vi "Configure Event Search.vi"   [LabVIEW 2010, in "Agilent 2000 3000 X-Series.lvlib"]
doc: "Configures the event search."
uses:
  <instrlib>/Agilent 2000 3000 X-Series/Agilent 2000 3000 X-Series.lvlib
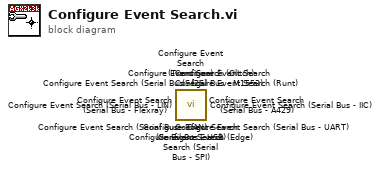
[diagram p0: block diagram]
diagram:
  n1 = call <instrlib>:"Configure Event Search (Serial Bus - USB).vi"() -> ()  [unwired: 10 in, 2 out]
  n2 = call <instrlib>:"Configure Event Search (Serial Bus - M1553).vi"() -> ()  [unwired: 10 in, 2 out]
  n3 = call <instrlib>:"Configure Event Search (Serial Bus - Flexray).vi"() -> ()  [unwired: 10 in, 2 out]
  n4 = call <instrlib>:"Configure Event Search (Serial Bus - A429).vi"() -> ()  [unwired: 10 in, 2 out]
  n5 = call <instrlib>:"Configure Event Search (Serial Bus - I2S).vi"() -> ()  [unwired: 10 in, 2 out]
  n6 = call <instrlib>:"Configure Event Search (Transition).vi"() -> ()  [unwired: 10 in, 2 out]
  n7 = call <instrlib>:"Configure Event Search (Serial Bus - UART).vi"() -> ()  [unwired: 10 in, 2 out]
  n8 = call <instrlib>:"Configure Event Search (Serial Bus - SPI).vi"() -> ()  [unwired: 10 in, 2 out]
  n9 = call <instrlib>:"Configure Event Search (Serial Bus - LIN).vi"() -> ()  [unwired: 10 in, 2 out]
  n10 = call <instrlib>:"Configure Event Search (Serial Bus - IIC).vi"() -> ()  [unwired: 10 in, 2 out]
  n11 = call <instrlib>:"Configure Event Search (Serial Bus - CAN).vi"() -> ()  [unwired: 10 in, 2 out]
  n12 = call <instrlib>:"Configure Event Search (Runt).vi"() -> ()  [unwired: 10 in, 2 out]
  n13 = call <instrlib>:"Configure Event Search (Glitch).vi"() -> ()  [unwired: 10 in, 2 out]
  n14 = call <instrlib>:"Configure Event Search (Edge).vi"() -> ()  [unwired: 10 in, 2 out]
